vi "Close LaunchPad.vi"(0 "VISA resource name":refnum<visa-resource-name>, 11 "error in":errorcluster) -> (15 "error out":errorcluster)   [LabVIEW 2015]
doc: "Closes the active connection to an Arduino."
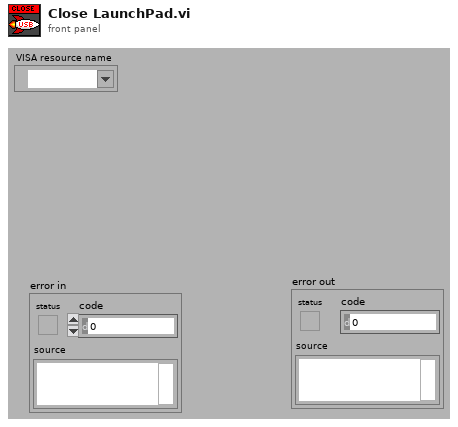
[diagram p1: front panel]
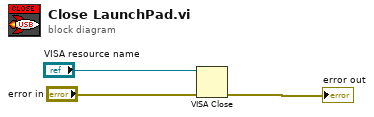
[diagram p0: block diagram]
diagram:
  n1 = VISA Close(VISA resource name="VISA resource name", error in (no error)="error in") -> (error out=→"error out":errorcluster)
